vi "consumer_loop.vi"(8 "error in (no error)":errorcluster, 10 "This VI":refnum<vi>, 11 "queue in":refnum<queue>) -> (0 "error out":errorcluster)   [LabVIEW 2020]
uses:
  controls/message cluster.ctl
  <instrlib>/Marlin Instrument Driver/Public/controls/axes.ctl
  <instrlib>/Marlin Instrument Driver/Public/controls/heater.ctl
  ea3af923-7d91-4754-a660-148973a20ef1.vi
  46caa509-a11f-4219-b2e3-e698adcdcc46.vi
  <vilib>/Utility/config.llb/NI_LVConfig.lvlib
  <instrlib>/Marlin Instrument Driver/Marlin Instrument Driver.lvlib
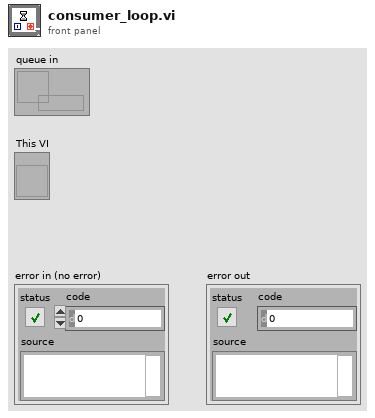
[diagram p1: front panel]
types:
  T1 = typedef "message cluster.ctl" = cluster{"message":string, "data":variant}
  T2 = typedef "NI_LVConfig.lvlib/Config Data RefNum.ctl" = refnum<k1>
  T3 = typedef "Marlin Instrument Driver.lvlib/axes.ctl" = cluster{"X":bool, "Y":bool, "Z":bool}
  T4 = typedef "Marlin Instrument Driver.lvlib/heater.ctl" = enum16{"Hot end", "Bed", "Chamber"}
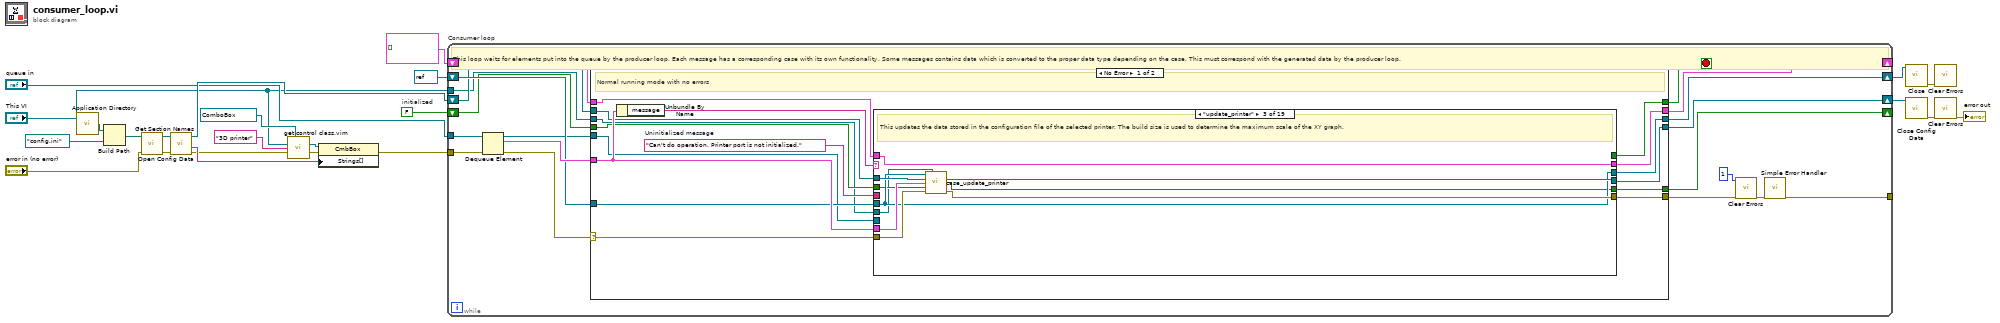
[diagram p0: block diagram]
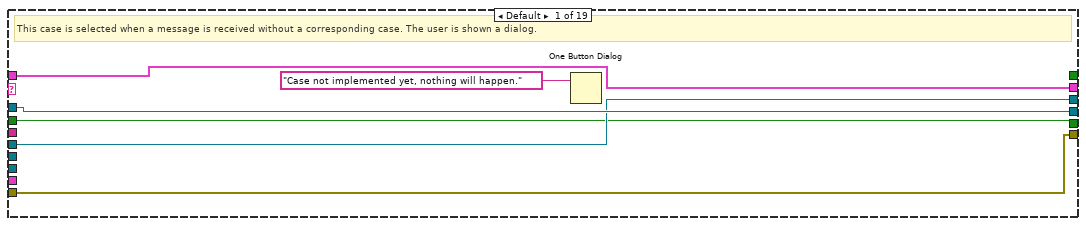
[diagram p2: hidden frame]
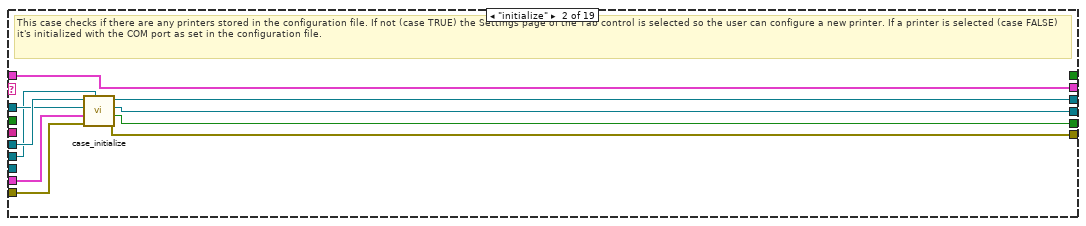
[diagram p3: hidden frame]
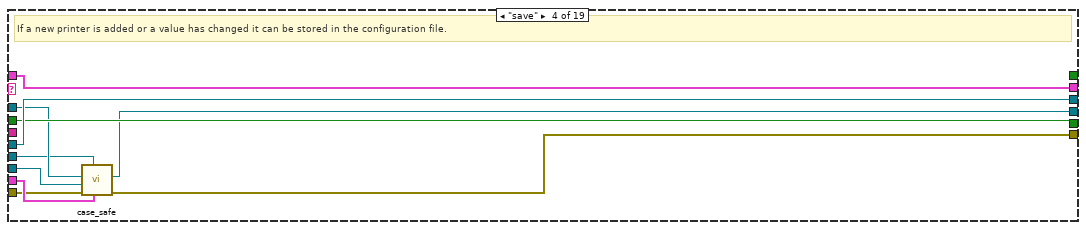
[diagram p4: hidden frame]
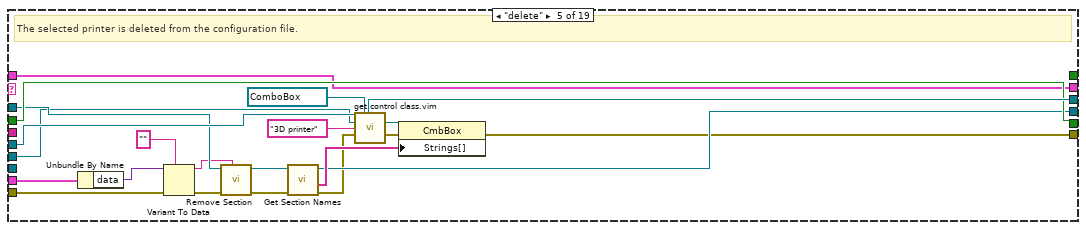
[diagram p5: hidden frame]
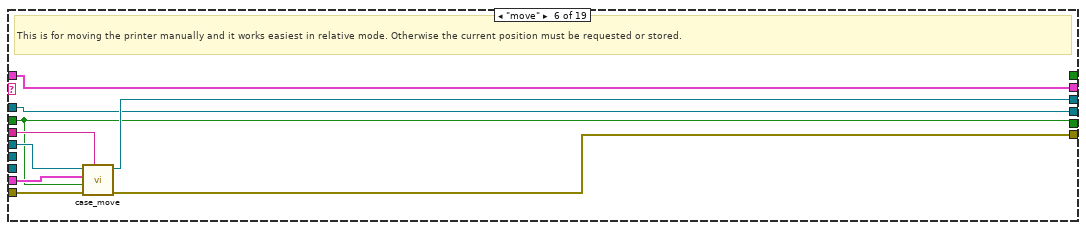
[diagram p6: hidden frame]
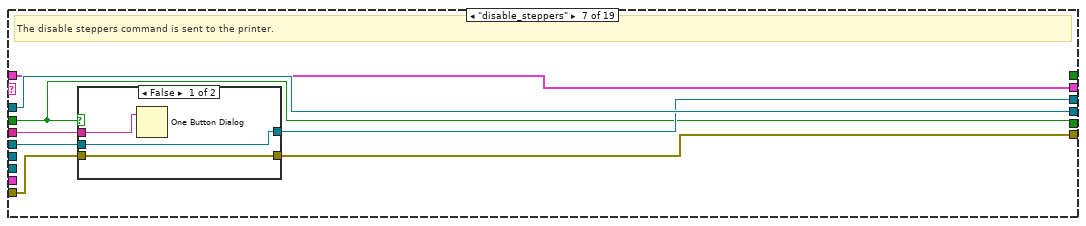
[diagram p7: hidden frame]
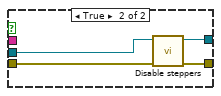
[diagram p8: hidden frame]
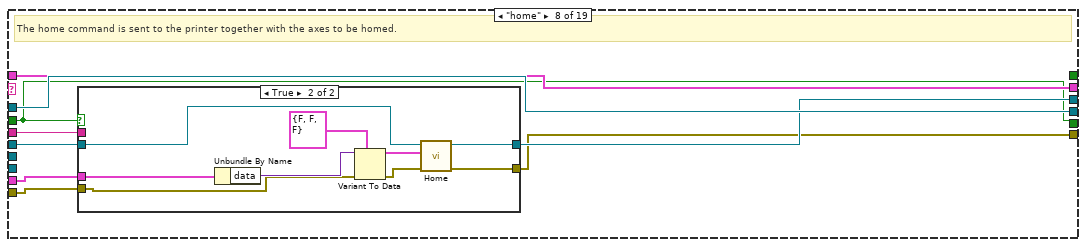
[diagram p9: hidden frame]
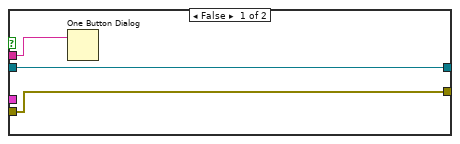
[diagram p10: hidden frame]
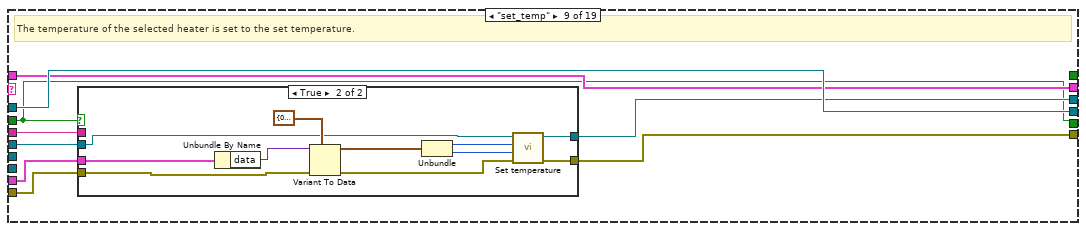
[diagram p11: hidden frame]
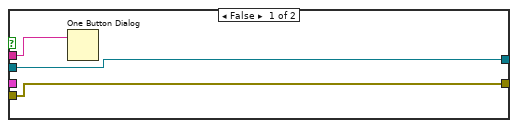
[diagram p12: hidden frame]
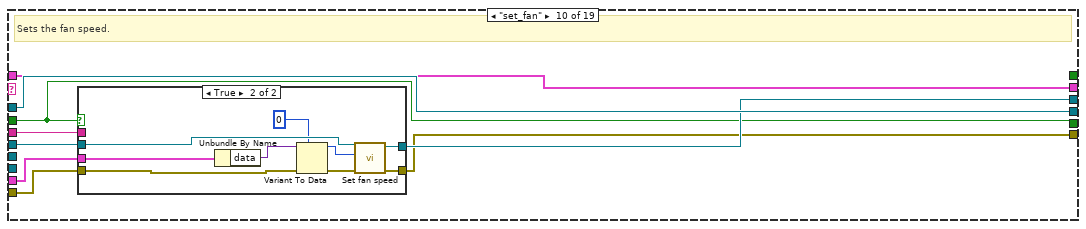
[diagram p13: hidden frame]
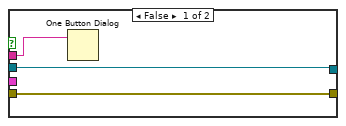
[diagram p14: hidden frame]
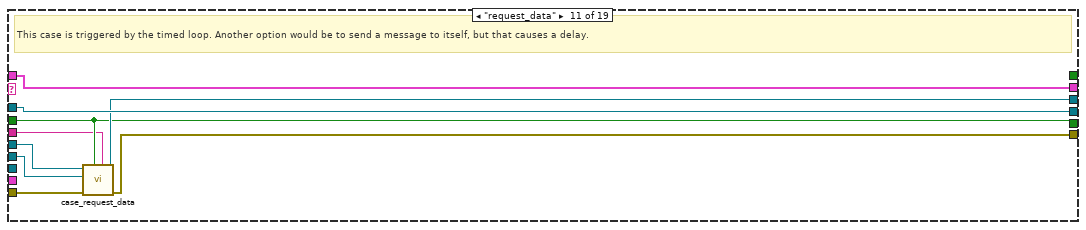
[diagram p15: hidden frame]
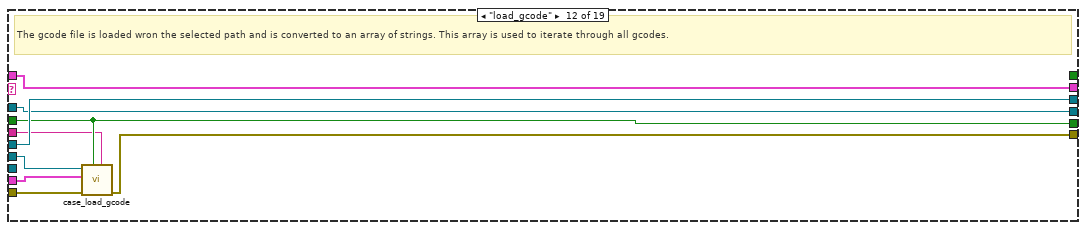
[diagram p16: hidden frame]
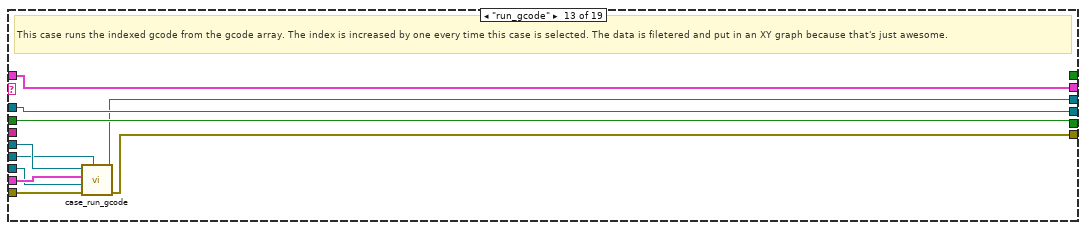
[diagram p17: hidden frame]
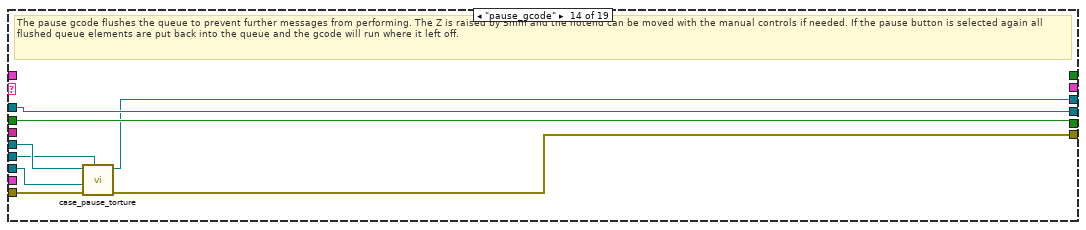
[diagram p18: hidden frame]
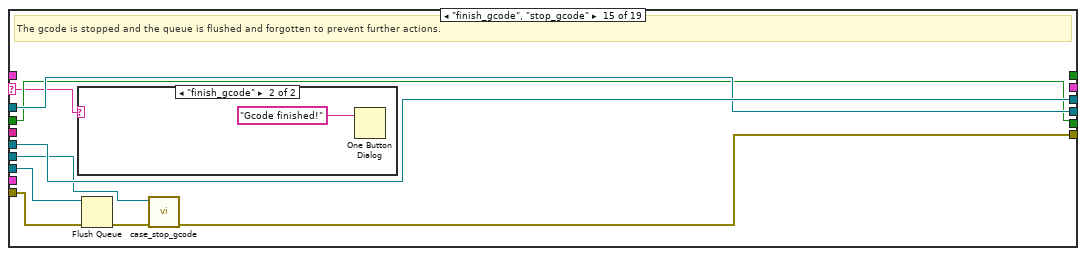
[diagram p19: hidden frame]
diagram:
  w8 = FALSE  # initialized
  n1 = call <vilib>:"Application Directory.vi"() -> ("Application Directory"=w9:path)
  n2 = Build Path(base path=w9, name or relative path=path "config.ini") -> (appended path=w11:path)
  n3 = call <vilib>:"Open Config Data.vi"("error in (no error)"="error in (no error)", "configuration file path"=w11) -> ("error out"=w16:errorcluster, "refnum"=w17:T2)  [unwired: 7 in, 1 out]
  n4 = call <vilib>:"Get Section Names.vi"("error in (no error)"=w16, "refnum"=w17) -> ("error out"=w3:errorcluster, "section names"=w20:string[], "refnum out"=w18:T2)  [unwired: 7 in]
  n5 = call "get control class.vim"("Control class"=refnum<vi> refnum ("reference out"), "Main VI reference"="This VI", "Label"="3D printer", "error in (no error)"=w3) -> ("Control out"=w4:refnum<vi>, "error out"=w2:errorcluster)  [unwired: 10 in]
  n6 = property on="Property Node" class="CmbBox"(reference=w4, error in=w2, "Strings[]"=w20) -> (error out=w19:errorcluster)  [unwired: 1 out]
  n7 = while "Consumer loop" {
    tunnel: "queue in" -> [w43]
    shift-right: [w38] -> w21
    shift-left: refnum<visa-resource-name> refnum ("VISA resource name out") -> [w36]
    shift-right: [w37] -> w13
    shift-left: w18 -> [w35]
    shift-right: [w34] -> _
    shift-left: w8 -> [w33]
    shift-right: [w28] -> _
    shift-left: T1[] [] ("remaining elements") -> [w27]
    tunnel: w19 -> [w39]
    tunnel: [w26] -> _
    tunnel: "This VI" -> [w25]
    stop <- w41 stop-if-true
    # "This loop waits for elements put into the queue by the producer loop. Each message has a corresponding case with its own functionality. Some messages contains data which is converted to the proper data type depending on the case. This must correspond with the generated data by the producer loop."
    n8 = Dequeue Element(queue=w43, error in (no error)=w39) -> (queue out=w32:refnum<queue>, element=w42:T1, error out=w40:errorcluster)  [unwired: 1 in, 1 out]
    n9 = case shown="No Error" w40 {
      selector: w40 -> [w56 _]
      tunnel: w42 -> [w58 _]
      tunnel: [w57 TRUE] -> w41
      tunnel: [w55 w287] -> w38
      tunnel: [w54 w286] -> w37
      tunnel: w36 -> [w53 w287]
      tunnel: w35 -> [w52 w286]
      tunnel: [w51 _] -> w34
      tunnel: w33 -> [w50 _]
      tunnel: w32 -> [w49 _]
      tunnel: [w48 _] -> w31
      tunnel: [w47 w284] -> w28
      tunnel: w27 -> [w46 w284]
      tunnel: w25 -> [w44 _]
      frame No Error {
        w45 = "Can't do operation. Printer port is not initialized."  # Uninitialized message
        # "Normal running mode with no errors"
        n10 = Unbundle By Name(w58) -> ("message"=w59:string)
        n11 = case shown="\"update_printer\"" w59 {
          selector: w59 -> [_ _ _ _ _ _ _ _ _ _ _ _ _ _ w242 _ _ _ _]
          tunnel: w58 -> [_ w68 w85 w91 w108 w125 _ w146 w168 w191 _ w217 w226 _ _ _ _ _ _]
          tunnel: [_ _ _ _ _ _ _ _ _ _ _ _ _ _ _ _ _ _ TRUE] -> w57
          tunnel: [w65 w75 w81 w88 w103 w124 w129 w144 w165 w188 w208 w219 w229 w237 w244 w256 w264 w271 w278] -> w48
          tunnel: w56 -> [w65 w73 w84 w89 w111 w123 w130 w147 w164 w187 w211 w221 w231 w238 w246 w258 w267 w272 w278]
          tunnel: [w63 w71 w80 w95 w116 w122 w128 w145 w166 w189 w213 w223 w230 w236 w250 w255 w265 w277 w279] -> w55
          tunnel: [w64 w70 w82 w87 w104 w121 w133 w149 w170 w193 w214 w222 w233 w241 w249 w261 w270 w276 w282] -> w54
          tunnel: w53 -> [w63 w69 w80 w95 w116 w120 w131 w148 w167 w190 w207 w223 w227 w235 w250 w259 w266 w277 w279]
          tunnel: w52 -> [w64 w67 w83 w92 w114 w121 w133 w149 w170 w193 w214 w222 w233 w241 w249 w261 w270 w276 w282]
          tunnel: [w62 w74 w76 w94 w115 w117 w126 w142 w163 w185 w210 w216 w232 w240 w248 w257 w269 w275 w281] -> w51
          tunnel: w50 -> [w62 _ w79 w94 w115 w117 w126 w142 w163 w185 w210 w216 w232 w240 w248 w257 w269 w275 w281]
          tunnel: w49 -> [_ _ _ w90 _ _ _ _ _ _ _ _ w225 w239 w247 w253 w262 w273 _]
          tunnel: [w61 w72 w78 w93 w102 w119 w132 w143 w169 w192 w212 w220 w228 _ _ w260 w268 w274 w280] -> w47
          tunnel: w46 -> [w61 w72 w78 w93 w102 w119 w132 w143 w169 w192 w212 w220 w228 _ _ w260 w268 w274 w280]
          tunnel: w45 -> [_ _ _ _ _ w118 w127 w141 w162 w186 w206 w215 _ _ _ w254 _ _ _]
          tunnel: w44 -> [_ w66 w77 w86 w99 _ _ _ _ _ w209 w218 w224 w234 w243 w252 w263 _ _]
          frame Default {
            # "This case is selected when a message is received without a corresponding case. The user is shown a dialog."
            n12 = One Button Dialog(message="Case not implemented yet, nothing will happen.") -> ()  [unwired: 1 in, 1 out]
          }
          frame "initialize" {
            # "This case checks if there are any printers stored in the configuration file. If not (case TRUE) the Settings page of the Tab control is selected so the user can configure a new printer. If a printer is selected (case FALSE) it's initialized with the COM port as set in the configuration file."
            n13 = call "case_initialize.vi"("Main VI reference"=w66, "error in (no error)"=w73, "message cluster"=w68, "Config refnum in"=w67, "VISA resource name in"=w69) -> ("error out"=w75:errorcluster, "initialized"=w74:bool, "Config refnum out"=w70:T2, "VISA resource name out"=w71:refnum<visa-resource-name>)  [unwired: 3 in]
          }
          frame "update_printer" {
            # "This updates the data stored in the configuration file of the selected printer. The build size is used to determine the maximum scale of the XY graph."
            n14 = call "case_update_printer.vi"("VISA resource name in"=w80, "Main VI reference"=w77, "Refnum in"=w83, "message cluster"=w85, "initialized"=w79, "error in (no error)"=w84) -> ("Refnum out"=w82:T2, "initialized out"=w76:bool, "error out"=w81:errorcluster)  [unwired: 7 in]
          }
          frame "save" {
            # "If a new printer is added or a value has changed it can be stored in the configuration file."
            n15 = call "case_safe.vi"("message cluster"=w91, "Main VI reference"=w86, "error in (no error)"=w89, "queue in"=w90, "config refnum in"=w92) -> ("error out"=w88:errorcluster, "config refnum out"=w87:T2)  [unwired: 5 in]
          }
          frame "delete" {
            # "The selected printer is deleted from the configuration file."
            n16 = Unbundle By Name(w108) -> ("data"=w113:variant)
            n17 = Variant To Data(error in=w111, type="", Variant=w113) -> (data=w109:string, error out=w110:errorcluster)
            n18 = call <vilib>:"Remove Section.vi"("section"=w109, "error in (no error)"=w110, "refnum"=w114) -> ("error out"=w105:errorcluster, "refnum out"=w106:T2)  [unwired: 6 in, 1 out]
            n19 = call <vilib>:"Get Section Names.vi"("error in (no error)"=w105, "refnum"=w106) -> ("error out"=w98:errorcluster, "section names"=w107:string[], "refnum out"=w104:T2)  [unwired: 7 in]
            n20 = call "get control class.vim"("Control class"=refnum<vi> refnum ("reference out"), "Main VI reference"=w99, "Label"="3D printer", "error in (no error)"=w98) -> ("Control out"=w96:refnum<vi>, "error out"=w97:errorcluster)  [unwired: 10 in]
            n21 = property on="Property Node" class="CmbBox"(reference=w96, error in=w97, "Strings[]"=w107) -> (error out=w103:errorcluster)  [unwired: 1 out]
          }
          frame "move" {
            # "This is for moving the printer manually and it works easiest in relative mode. Otherwise the current position must be requested or stored."
            n22 = call "case_move.vi"("Uninitialized message"=w118, "error in (no error)"=w123, "initialized"=w117, "message cluster"=w125, "VISA Refnum in"=w120) -> ("error out"=w124:errorcluster, "VISA Refnum out"=w122:refnum<visa-resource-name>)  [unwired: 5 in]
          }
          frame "disable_steppers" {
            # "The disable steppers command is sent to the printer."
            n23 = case shown="False" w126 {
              tunnel: w131 -> [w136 w140]
              tunnel: w130 -> [w135 w139]
              tunnel: [w135 w138] -> w129
              tunnel: [w136 w137] -> w128
              tunnel: w127 -> [w134 _]
              frame False {
                n24 = One Button Dialog(message=w134) -> ()  [unwired: 1 in, 1 out]
              }
              frame True {
                n25 = call <instrlib>:"Disable steppers.vi"("error in (no error)"=w139, "VISA resource name"=w140) -> ("error out"=w138:errorcluster, "VISA resource name out"=w137:refnum<visa-resource-name>)  [unwired: 8 in]
              }
            }
          }
          frame "home" {
            # "The home command is sent to the printer together with the axes to be homed."
            n26 = case shown="True" w142 {
              tunnel: w148 -> [w151 w161]
              tunnel: w147 -> [w150 w159]
              tunnel: w146 -> [_ w158]
              tunnel: [w151 w154] -> w145
              tunnel: [w150 w153] -> w144
              tunnel: w141 -> [w152 _]
              frame False {
                n27 = One Button Dialog(message=w152) -> ()  [unwired: 1 in, 1 out]
              }
              frame True {
                n28 = Unbundle By Name(w158) -> ("data"=w160:variant)
                n29 = Variant To Data(error in=w159, type=T3 {"X"=FALSE, "Y"=FALSE, "Z"=FALSE} ("Axes"), Variant=w160) -> (data=w156:T3, error out=w155:errorcluster)
                n30 = call <instrlib>:"Home.vi"("error in (no error)"=w155, "Axes"=w156, "VISA resource name"=w161) -> ("error out"=w153:errorcluster, "VISA resource name out"=w154:refnum<visa-resource-name>)  [unwired: 7 in]
              }
            }
          }
          frame "set_temp" {
            # "The temperature of the selected heater is set to the set temperature."
            n31 = case shown="True" w163 {
              tunnel: w168 -> [_ w184]
              tunnel: w167 -> [w171 w178]
              tunnel: [w171 w177] -> w166
              tunnel: [w172 w176] -> w165
              tunnel: w164 -> [w172 w175]
              tunnel: w162 -> [w173 _]
              frame False {
                n32 = One Button Dialog(message=w173) -> ()  [unwired: 1 in, 1 out]
              }
              frame True {
                n33 = Unbundle By Name(w184) -> ("data"=w183:variant)
                n34 = Variant To Data(error in=w175, type=cluster{"setpoint":i32, "Heater":T4} {"setpoint"=0, "Heater"=enum."Hot end"} ("output cluster"), Variant=w183) -> (data=w181:cluster{"setpoint":i32, "Heater":T4}, error out=w174:errorcluster)
                n35 = Unbundle(w181) -> ("setpoint"=w180:i32, "Heater"=w179:T4)
                n36 = call <instrlib>:"Set temperature.vi"("error in (no error)"=w174, "Heater"=w179, "Temperature"=w180, "VISA resource name"=w178) -> ("error out"=w176:errorcluster, "VISA resource name out"=w177:refnum<visa-resource-name>)  [unwired: 6 in]
              }
            }
          }
          frame "set_fan" {
            # "Sets the fan speed."
            n37 = case shown="True" w185 {
              tunnel: w191 -> [_ w205]
              tunnel: w190 -> [w194 w203]
              tunnel: [w194 w202] -> w189
              tunnel: [w195 w201] -> w188
              tunnel: w187 -> [w195 w200]
              tunnel: w186 -> [w196 _]
              frame False {
                n38 = One Button Dialog(message=w196) -> ()  [unwired: 1 in, 1 out]
              }
              frame True {
                n39 = Unbundle By Name(w205) -> ("data"=w204:variant)
                n40 = Variant To Data(error in=w200, type=u8 0 ("Fan speed"), Variant=w204) -> (data=w197:u8, error out=w199:errorcluster)
                n41 = call <instrlib>:"Set fan speed.vi"("error in (no error)"=w199, "Fan speed"=w197, "VISA resource name"=w203) -> ("error out"=w201:errorcluster, "VISA resource name out"=w202:refnum<visa-resource-name>)  [unwired: 7 in]
              }
            }
          }
          frame "request_data" {
            # "This case is triggered by the timed loop. Another option would be to send a message to itself, but that causes a delay."
            n42 = call "case_request_data.vi"("Uninitialized message"=w206, "initialized"=w210, "error in (no error)"=w211, "This VI"=w209, "VISA resource name in"=w207) -> ("error out"=w208:errorcluster, "VISA Refnum out"=w213:refnum<visa-resource-name>)  [unwired: 5 in]
          }
          frame "load_gcode" {
            # "The gcode file is loaded wron the selected path and is converted to an array of strings. This array is used to iterate through all gcodes."
            n43 = call "case_load_gcode.vi"("Uninitialized message"=w215, "initialized"=w216, "error in (no error)"=w221, "message cluster"=w217, "Main VI reference"=w218) -> ("error out"=w219:errorcluster)  [unwired: 6 in]
          }
          frame "run_gcode" {
            # "This case runs the indexed gcode from the gcode array. The index is increased by one every time this case is selected. The data is filetered and put in an XY graph because that's just awesome."
            n44 = call "case_run_gcode.vi"("Main VI reference"=w224, "error in (no error)"=w231, "queue in"=w225, "message cluster"=w226, "VISA resource name in"=w227) -> ("error out"=w229:errorcluster, "VISA Refnum out"=w230:refnum<visa-resource-name>)  [unwired: 5 in]
          }
          frame "pause_gcode" {
            # "The pause gcode flushes the queue to prevent further messages from performing. The Z is raised by 5mm and the hotend can be moved with the manual controls if needed. If the pause button is selected again all flushed queue elements are put back into the queue and the gcode will run where it left off."
            n45 = call "case_pause_torture.vi"("Main VI reference"=w234, "error in (no error)"=w238, "queue in"=w239, "VISA resource name in"=w235) -> ("error out"=w237:errorcluster, "VISA Refnum out"=w236:refnum<visa-resource-name>)  [unwired: 6 in]
          }
          frame "finish_gcode", "stop_gcode" {
            # "The gcode is stopped and the queue is flushed and forgotten to prevent further actions."
            n46 = case shown="\"finish_gcode\"" w242 {
              frame Default {
              }
              frame "finish_gcode" {
                n47 = One Button Dialog(message="Gcode finished!") -> ()  [unwired: 1 in, 1 out]
              }
            }
            n48 = Flush Queue(queue=w247, error in (no error)=w246) -> (error out=w245:errorcluster)  [unwired: 2 out]
            n49 = call "case_stop_gcode.vi"("error in (no error)"=w245, "VI in"=w243) -> ("error out"=w244:errorcluster)  [unwired: 9 in]
          }
          frame "start_torture" {
            # "The torture sequence is started. The printer is homed after which the head is placed into the center at a Z height of 10mm. The torture sequence is selected."
            n50 = call "case_start_torture.vi"("Uninitialized message"=w254, "initialized"=w257, "error in (no error)"=w258, "Main VI reference"=w252, "queue in"=w253, "VISA Refnum in"=w259) -> ("error out"=w256:errorcluster, "VISA Refnum out"=w255:refnum<visa-resource-name>)  [unwired: 4 in]
          }
          frame "torture" {
            # "This sequence moves the print head symmetric from the bed center back and forth without waiting. The frequence can be changed by changing the travel distance or movement speed. This case calls itself to stay in a loop."
            n51 = call "case_torture.vi"("Main VI reference"=w263, "error in (no error)"=w267, "queue in"=w262, "VISA resource name in"=w266) -> ("error out"=w264:errorcluster, "VISA Refnum out"=w265:refnum<visa-resource-name>)  [unwired: 6 in]
          }
          frame "stop_torture" {
            # "The queue is flushed so the remaining torture messages aren't performed anymore."
            n52 = Flush Queue(queue=w273, error in (no error)=w272) -> (error out=w271:errorcluster)  [unwired: 2 out]
          }
          frame "close" {
            # "This closes the port and ends the loop."
          }
        }
      }
      frame Error {
        # "This case is selected when the Dequeue element generates an error. This means that the queue is released and this loop is stopped."
      }
    }
    n53 = call <vilib>:"Clear Errors.vi"("error in (no error)"=w31, "specific error code to clear (0: all)"=1) -> ("error out"=w30:errorcluster)  [unwired: 4 in, 1 out]
    n54 = call <vilib>:"Simple Error Handler.vi"("error in (no error)"=w30) -> ("error out"=w26:errorcluster)  [unwired: 4 in, 4 out]
  }
  n55 = call <instrlib>:"Close.vi"("VISA resource name"=w21) -> ("error out"=w22:errorcluster)  [unwired: 10 in]
  n56 = call <vilib>:"Close Config Data.vi"("refnum"=w13) -> ("error out"=w23:errorcluster)  [unwired: 9 in, 1 out]
  n57 = call <vilib>:"Clear Errors.vi"("error in (no error)"=w22) -> ()  [unwired: 5 in, 2 out]
  n58 = call <vilib>:"Clear Errors.vi"("error in (no error)"=w23) -> ("error out"=→"error out":errorcluster)  [unwired: 5 in, 1 out]
